vi "Write IODevInfo.vi"(8 "error in (no error)":errorcluster, 10 "IODevInfo.lvclass":refnum<class "IODevInfo.lvclass">, 11 "IO Device in":refnum<class "IO Device.lvclass">) -> (0 "error out":errorcluster, 3 "IO Device out":refnum<class "IO Device.lvclass">)   [LabVIEW 2015, in "IO Device.lvlib" / "IO Device.lvclass"]
uses:
  IO Device.lvclass
  IODevInfo.lvclass
  IO Device.lvclass/IO Device.ctl
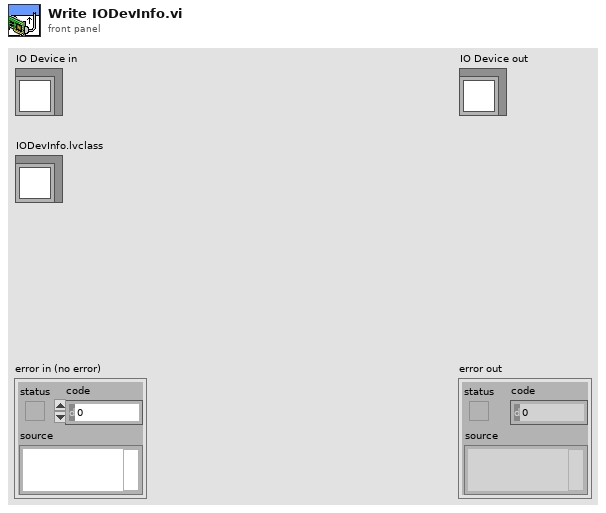
[diagram p1: front panel]
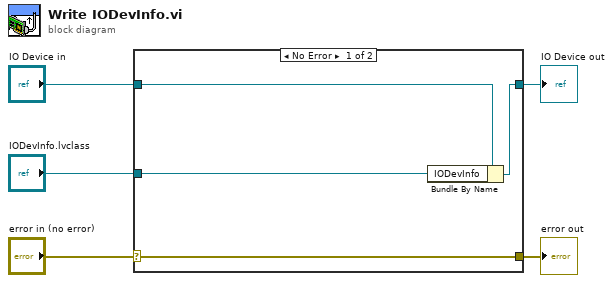
[diagram p0: block diagram]
diagram:
  n1 = case shown="No Error" "error in (no error)" {
    selector: "error in (no error)" -> [w9 w10]
    tunnel: [w9 w10] -> w4
    tunnel: [w7 w11] -> w2
    tunnel: "IO Device in" -> [w8 w11]
    tunnel: "IODevInfo.lvclass" -> [w6 _]
    frame No Error {
      n2 = Bundle By Name(cluster=w8, "IODevInfo"=w6) -> (w7:refnum<class "IO Device.lvclass">)
    }
    frame Error {
    }
  }
  "error out" <- w4
  "IO Device out" <- w2
